vi "RT Driver VI.vi"(7 "Operation":T1, 11 "Device Reference in":T2 format="%.0x") -> (0 "Error Code":i32)   [LabVIEW 2020, in "FPGA Addon Engine.lvlib"]
uses:
  FPGA Addon Engine.lvlib
  <vilib>/NI VeriStand/Custom Device API/Custom Device Item Ref.ctl
  <vilib>/NI VeriStand/Custom Device API/Hardware Interface Driver VI Operation.ctl
  <vilib>/NI/NIVS Inline Async API/_VS Inline Async API/VS Inline Async API/Types/Error Handling Settings.ctl
  <vilib>/NI/NIVS Inline Async API/_VS Inline Async API/VS Inline Async API/VS Inline Async API.lvclass/VS Inline Async API.ctl
  <vilib>/NI/NIVS Inline Async API/_Data Access Engine/Data Access Engine/Data Access Engine.lvclass/Data Access Engine.ctl
  <vilib>/NI/NIVS Inline Async API/_Data Access Engine/Access Type Classes/Write/Write.lvclass/Write.ctl
  <vilib>/NI/NIVS Inline Async API/_Data Access Engine/Access Type Classes/ReadWrite/ReadWrite.lvclass/ReadWrite.ctl
  Addon Shared/SubVIs/FPGA Settings.vi
  SubVIs/Initialize Scalar Datatypes and Refs.vi
  <vilib>/NI/NIVS Inline Async API/_Data Access Engine/Data Access Engine/Methods/Data.Engine.Read Data from HW.vi
  <vilib>/NI/NIVS Inline Async API/_VS Inline Async API/Error Handling Process/SubVIs/Error.GetError.vi
  <vilib>/NI/NIVS Inline Async API/_Data Access Engine/Access Type Classes/ReadWrite/ReadWrite.EngineData.vi
  <vilib>/NI/NIVS Inline Async API/_Data Access Engine/Access Type Classes/Write/Write.EngineData.vi
  <vilib>/NI VeriStand/Custom Device API/NI VeriStand - Get Channel Value by Data Reference.vi
  <vilib>/NI VeriStand/Custom Device API/NI VeriStand - Set Channel Value by Data Reference.vi
  <vilib>/Utility/config.llb/Open Config Data.vi
  <vilib>/Utility/config.llb/Get Key Names.vi
  <vilib>/Utility/config.llb/Write Key.vi
  <vilib>/Utility/config.llb/Write Key (I32).vi
  <vilib>/Utility/config.llb/Close Config Data.vi
  Addon Shared/SubVIs/Constants.vi
  <vilib>/NI VeriStand/Custom Device API/NI VeriStand - Get Item Property.vi
  <vilib>/NI VeriStand/Custom Device API/Get Item Property (Variant).vi
  <vilib>/NI VeriStand/Custom Device API/Get Item Property (Dependent File).vi
  <vilib>/NI VeriStand/Custom Device API/Get Item Property (Path).vi
  <vilib>/NI VeriStand/Custom Device API/Get Item Property (String).vi
  <vilib>/NI VeriStand/Custom Device API/Get Item Property (Boolean).vi
  <vilib>/NI VeriStand/Custom Device API/NI VeriStand - Set Item Property.vi
  <vilib>/NI VeriStand/Custom Device API/Set Item Property (Path).vi
  <vilib>/NI VeriStand/Custom Device API/Set Item Property (String).vi
  <vilib>/NI VeriStand/Custom Device API/Set Item Property (Boolean).vi
  APIs/FPGA Register IO/Utilities/Open FPGA Session.vi
  SubVIs/Initialize Input DMA Refs.vi
  SubVIs/Initialize Output DMA Refs.vi
  SubVIs/Initialize Scalar Datatype Classes.vi
  <vilib>/Utility/SystemLogging/Write to System Log.vi
  <vilib>/Utility/error.llb/Error Cluster From Error Code.vi
  <vilib>/RVI Host/nirviSupport.llb/nirviErrorClusterFromErrorCode.vi
  <vilib>/rvi/errors/niLvFpgaAdjustHostInterfaceError.vi
  <vilib>/NI VeriStand/Custom Device API/Global Data Refs.vi
  <vilib>/FPGAPlugInAG/Dynamic/niLvFpga_Close_Dynamic.vi
  <vilib>/NI VeriStand/Custom Device Waveform API/Multiple Waveforms Write (DBL)/Multiple Waveforms Write (DBL).lvclass
  <vilib>/NI VeriStand/Custom Device Waveform API/Single Waveform Read (DBL)/Single Waveform Read (DBL).lvclass
  <vilib>/NI/NIVS Inline Async API/_VS Inline Async API/VS Inline Async API/VS Inline Async API.lvclass
  <vilib>/rvi/interface/nirviMethod/nirviMethod.xnode
  <vilib>/rvi/interface/nirviCloseFPGA/nirviCloseFPGA.xnode
  <vilib>/NI VeriStand/Custom Device API/Custom Device API.lvlib
  <vilib>/rvi/interface/nirviMethod/StockFPGA_InlinedMethodWaitForSingleIRQ.vi
  <vilib>/FPGAPlugInAG/Dynamic/niLvFpga_WaitOnIrq_Dynamic.vi
  <vilib>/FPGAPlugInAG/Dynamic/niLvFpga_AcknowledgeIrq_Dynamic.vi
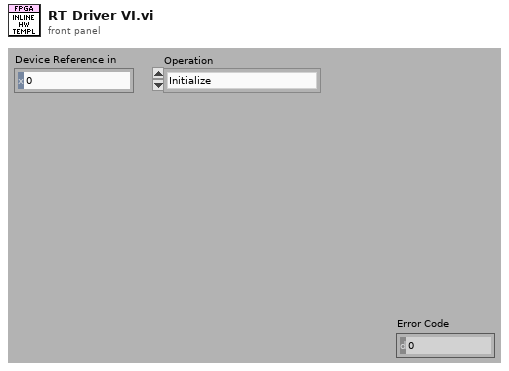
[diagram p1: front panel]
types:
  T1 = typedef "Custom Device API.lvlib/Hardware Interface Driver VI Operation.ctl" = enum16{"Initialize", "Start", "Read Data from HW", "Write Data to HW", "Close"}
  T2 = typedef "Custom Device API.lvlib/Custom Device Item Ref.ctl" = u64
  T3 = typedef "FPGA Addon Engine.lvlib/State Variables.ctl" = cluster{"FPGA Ref":refnum<k20>, "IncomingRegisters.Refs":T4[], "IncomingDMA.Refs":T7[], "OutgoingRegisters.Refs":T4[], "OutgoingDMA.Refs":T12[], "Compiled":T14}
  T4 = typedef "FPGA Addon Engine.lvlib/Register Settings.ctl" = cluster{"Name":string, "Data Type":T5, "session":u32, "Scalar Type":T6, "Index":i32, "Length":i32, "attributes":variant, "default value":variant}
  T5 = typedef "FPGA Addon Shared.lvlib/FPGA Addon Data Type.ctl" = enum8{"<Null>", "I8", "I16", "I32", "I64", "U8", "U16", "U32", "U64", "SGL", "Boolean", "Analog PWM In Settings", "Analog PWM In", "Digital PWM In Settings", "Digital PWM In", "Digital PWM Out", "Sine Out", "FXP", "FXP+/-24.5", "FXP+/-16.5", "FXP+/-32.8", "FXP+/-64.32", "FXP+/-16.7", "FXP+/-20.5", "FXP+/-27.5", "FXP+/-32.16", "FXP+16.3", "FXP+18.3", "Digital Static In", "Digital Static Out", "Digital Static In Settings", "Digital WSS Out", "Quad Encoder Settings", "Quad Encoder In", "Group"}
  T6 = typedef "FPGA Addon Shared.lvlib/Scalar Type.ctl" = enum16{"Standard", "Bitpacked"}
  T7 = typedef "FPGA Addon Engine.lvlib/DMA Input References.ctl" = cluster{"Addon Name":string, "Waveform Ref":refnum<class "Multiple Waveforms Write (DBL).lvclass">, "DMA Name":string, "DMA Settings":T8, "Refs":T11}
  T8 = typedef "FPGA Addon Shared.lvlib/DMA Settings.ctl" = cluster{"Number of Channels":u8, "Delacing Scheme":T9, "Update Rate":u32, "dt":dbl, "Mode":T10, "Number of Samples":u32, "DMA Host Buffer":u32}
  T9 = typedef "FPGA Addon Shared.lvlib/Delacing Scheme.ctl" = enum8{"Interleaved", "Bitpacked"}
  T10 = typedef "FPGA Addon Shared.lvlib/DMA Acquisition Mode.ctl" = enum8{"Continuous", "Triggered Finite"}
  T11 = typedef "FPGA Addon Engine.lvlib/DMA Input Refs.ctl" = cluster{"Data Type":T5, "DMA_SGL":refnum<k20>, "DMA_U64":refnum<k20>, "DMA_I64":refnum<k20>, "DMA_FXP+/-32.8":refnum<k20>, "DMA_FXP+/-64.32":refnum<k20>, "DMA_U32":refnum<k20>, "DMA_U16":refnum<k20>, "DMA_U8":refnum<k20>, "DMA_I32":refnum<k20>, "DMA_I16":refnum<k20>, "DMA_I8":refnum<k20>, "DMA_FXP+/-32.16":refnum<k20>}
  T12 = typedef "FPGA Addon Engine.lvlib/DMA Output References.ctl" = cluster{"Addon Name":string, "Waveforms":refnum<class "Single Waveform Read (DBL).lvclass">[], "DMA Name":string, "Refs":T13}
  T13 = typedef "FPGA Addon Engine.lvlib/DMA Output Refs.ctl" = cluster{"Data Type":T5, "DMA_SGL":refnum<k20>, "DMA_U64":refnum<k20>, "DMA_I64":refnum<k20>, "DMA_FXP+/-32.8":refnum<k20>, "DMA_FXP+/-64.32":refnum<k20>, "DMA_U32":refnum<k20>, "DMA_U16":refnum<k20>, "DMA_U8":refnum<k20>, "DMA_I32":refnum<k20>, "DMA_I16":refnum<k20>, "DMA_I8":refnum<k20>, "DMA_FXP+/-32.16":refnum<k20>}
  T14 = typedef "FPGA Addon Shared.lvlib/Compiled.Settings.ctl" = cluster{"Name":string, "IncomingRegisters.Settings":T15[], "IncomingRegisters.Refs":cluster{"Refs":T17[], "Values":dbl[]}, "OutgoingRegisters.Settings":T15[], "OutgoingRegisters.Refs":cluster{"Refs":T17[], "Values":dbl[]}, "Incoming.Size":i32, "Outgoing.Size":i32, "IncomingDMA.Settings":T19[], "OutgoingDMA.Settings":T19[], "FPGA.Settings":T21, "Target.Type":T22}
  T15 = typedef "FPGA Addon Shared.lvlib/Compiled.RegisterSettings.ctl" = cluster{"Scalar Type":T6, "Index":i32, "Length":i32, "Register":T16}
  T16 = typedef "FPGA Addon Shared.lvlib/Register Information.ctl" = cluster{"Name":string, "Data Type":T5, "Default Value":variant, "Attributes":variant}
  T17 = typedef "Custom Device API.lvlib/Block Data Reference.ctl" = cluster{"Data Reference":T18, "Offset":u64, "Length":u64}
  T18 = typedef "Custom Device API.lvlib/Data Reference.ctl" = i32
  T19 = typedef "FPGA Addon Shared.lvlib/Compiled.DMASettings.ctl" = cluster{"Name":string, "Data Type":T5, "DMA.Settings":T8, "DMA.VSRefs":T20[]}
  T20 = typedef "Custom Device API.lvlib/Waveform Data Reference.ctl" = i32
  T21 = typedef "FPGA Addon Shared.lvlib/FPGA Settings.ctl" = cluster{"Bitfile path":path, "RIO Device Address":string, "Group":bool}
  T22 = typedef "Custom Device API.lvlib/Custom Device Target Type.ctl" = enum16{"PharLap", "VxWorks", "Windows", "Linux_32_ARM", "Linux_x64"}
  T23 = cluster{"Vars":T3, "Async?":bool, "Async":refnum<class "VS Inline Async API.lvclass">}
  T24 = typedef "VS Inline Async API.lvlib/VS Inline Async API.lvclass/Error Handling Settings.ctl" = cluster{"Write to SystemLog (F)":bool}
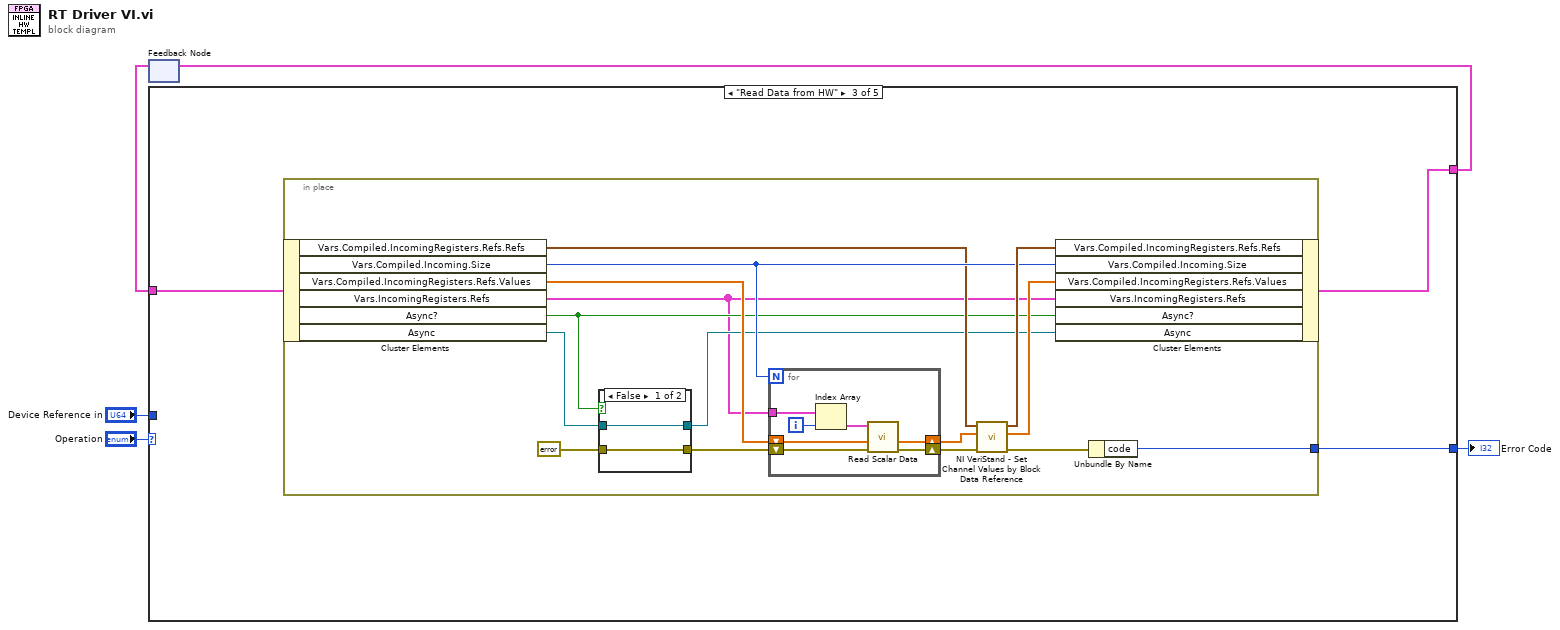
[diagram p0: block diagram]
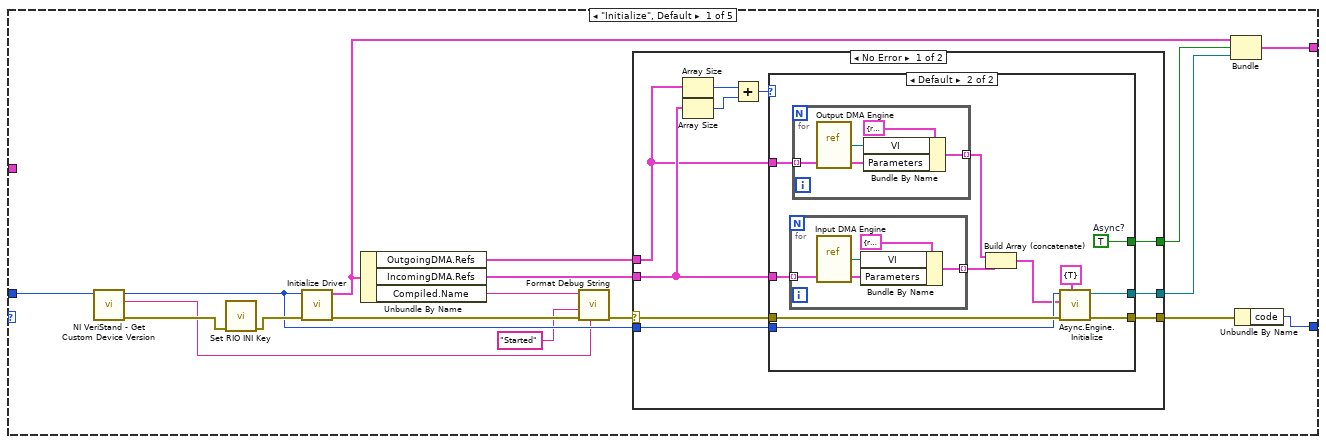
[diagram p2: hidden frame]
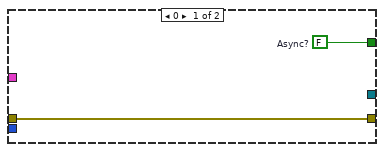
[diagram p3: hidden frame]
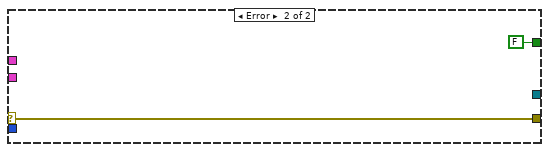
[diagram p4: hidden frame]
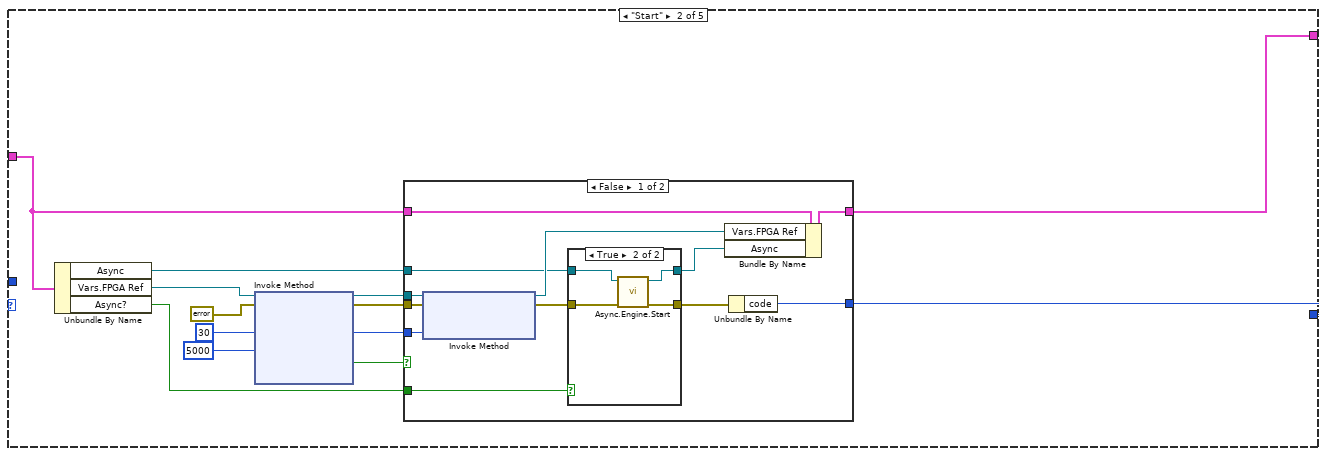
[diagram p5: hidden frame]
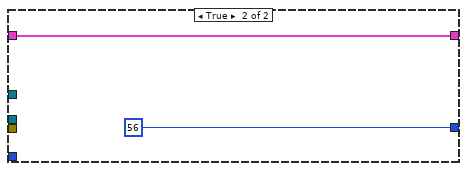
[diagram p7: hidden frame]
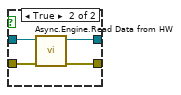
[diagram p8: hidden frame]
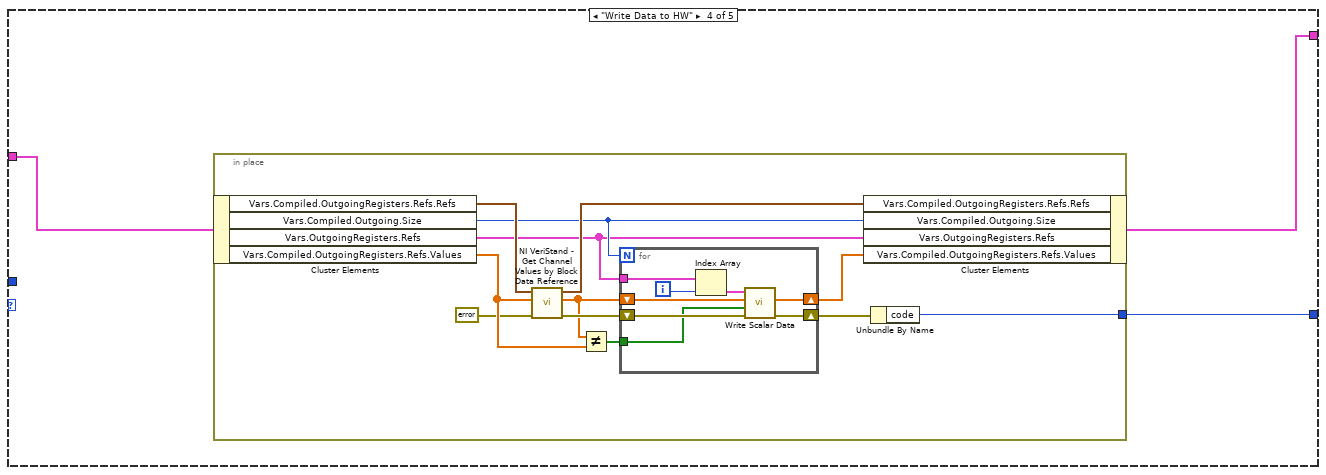
[diagram p9: hidden frame]
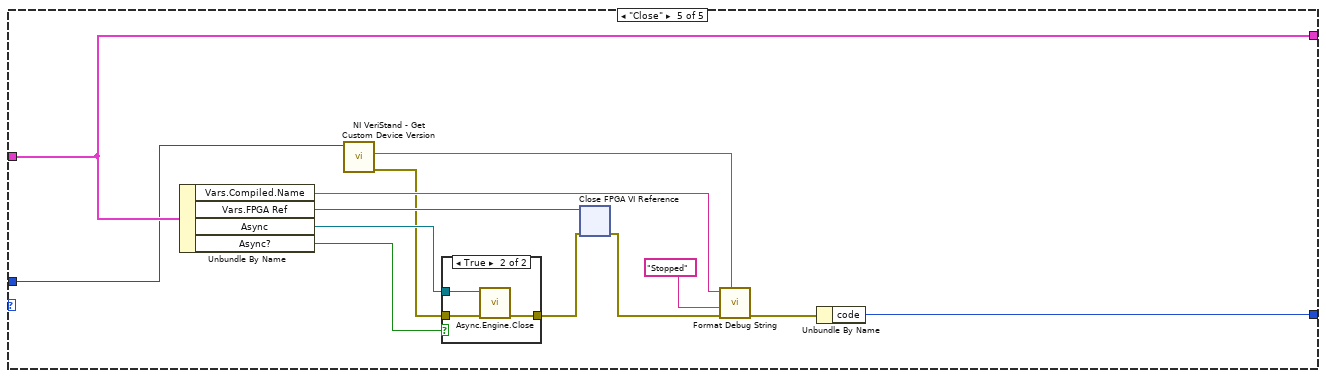
[diagram p10: hidden frame]
diagram:
  n1 = feedback #1() -> (w3:T23)  [unwired: 1 out]
  n2 = case shown="\"Read Data from HW\"" "Operation" {
    tunnel: [w22 w65 w90 w120 w153] -> w4
    tunnel: w3 -> [_ w66 w88 w121 w153]
    tunnel: "Device Reference in" -> [w12 _ _ _ w148]
    tunnel: [w21 w67 w89 w119 w154] -> w1
    frame "Initialize", Default {
      n3 = call <vilib>:"NI VeriStand - Get Custom Device Version.vi"("Device Ref in"=w12) -> ("error out"=w13:errorcluster, "Value"=w9:string, "Device Ref out"=w11:T2)  [unwired: 8 in]
      n4 = call "Set RIO INI Key.vi"("error in (no error)"=w13) -> ("error out"=w20:errorcluster)  [unwired: 10 in]
      n5 = call "Initialize Driver.vi"("error in (no error)"=w20, "Section Ref in"=w11) -> ("error out"=w10:errorcluster, "Vars"=w14:T3)  [unwired: 8 in]
      n6 = Unbundle By Name(w14) -> ("OutgoingDMA.Refs"=w16:T12[], "IncomingDMA.Refs"=w17:T7[], "Compiled.Name"=w8:string)
      n7 = call "Format Debug String.vi"("Version"=w9, "error in (no error)"=w10, "State"="Started" ("string"), "Name"=w8) -> ("error out"=w6:errorcluster)  [unwired: 7 in]
      n8 = case shown="No Error" w6 {
        selector: w6 -> [w23 w55]
        tunnel: [w32 w55] -> w19
        tunnel: [w31 _] -> w18
        tunnel: w17 -> [w30 _]
        tunnel: w16 -> [w29 _]
        tunnel: [w25 FALSE ("Async?")] -> w15
        tunnel: w11 -> [w24 _]
        frame No Error {
          n9 = Array Size(array=w29) -> (size(s)=w28:i32)
          n10 = Array Size(array=w30) -> (size(s)=w27:i32)
          n11 = Add(x=w28, y=w27) -> (x+y=w26:i32)
          n12 = case shown="Default" w26 {
            tunnel: w23 -> [w34 w42]
            tunnel: [w34 w41] -> w32
            tunnel: [_ w40] -> w31
            tunnel: w30 -> [_ w38]
            tunnel: w29 -> [_ w45]
            tunnel: [w33 w43] -> w25
            tunnel: w24 -> [_ w39]
            frame 0 {
              w33 = FALSE  # Async?
            }
            frame Default {
              w43 = TRUE  # Async?
              n13 = for {
                tunnel: w38 -> [w46] mode=indexing
                tunnel: [w48] -> w37 mode=indexing
                n14 = vi-ref "Input DMA Engine.vi"() -> (w47:refnum<vi>)
                n15 = Bundle By Name(cluster=cluster{"VI":refnum<vi>, "Parameters":variant} {"VI"=refnum, "Parameters"=variant} ("Process"), "VI"=w47, "Parameters"=w46) -> (w48:cluster{"VI":refnum<vi>, "Parameters":variant})
              }
              n16 = for {
                tunnel: w45 -> [w52] mode=indexing
                tunnel: [w51] -> w44 mode=indexing
                n17 = vi-ref "Output DMA Engine.vi"() -> (w50:refnum<vi>)
                n18 = Bundle By Name(cluster=cluster{"VI":refnum<vi>, "Parameters":variant} {"VI"=refnum, "Parameters"=variant} ("Process"), "VI"=w50, "Parameters"=w52) -> (w51:cluster{"VI":refnum<vi>, "Parameters":variant})
              }
              n19 = Build Array (concatenate)(w44, w37) -> (w36:cluster{"VI":refnum<vi>, "Parameters":variant}[])
              n20 = call <vilib>:"Async.Engine.Initialize.vi"("Error Log Settings"=T24 {"Write to SystemLog (F)"=TRUE}, "error in (no error)"=w42, "Processes"=w36, "Custom Device Ref"=w39) -> ("error out"=w41:errorcluster, "Async"=w40:refnum<class "VS Inline Async API.lvclass">)  [unwired: 6 in]
            }
          }
        }
        frame Error {
        }
      }
      n21 = Bundle("Vars"=w14, "Async?"=w15, "Async"=w18) -> (w22:T23)  [unwired: 1 out]
      n22 = Unbundle By Name(w19) -> ("code"=w21:i32)
    }
    frame "Start" {
      w61 = 30 ("IRQ Number(s)")
      n23 = Unbundle By Name(w66) -> ("Async"=w57:refnum<class "VS Inline Async API.lvclass">, "Vars.FPGA Ref"=w64:refnum<k20>, "Async?"=w59:bool)
      n24 = xnode "Invoke Method"("FPGA VI Reference In"=w64, "error in"=errorcluster {"status"=FALSE, "code"=0, "source"=""}, "IRQ Number(s)"=w61, "Timeout (ms)"=5000) -> ("FPGA VI Reference Out"=w63:refnum<k20>, "error out"=w62:errorcluster, "Timed Out"=w58:bool)  [unwired: 1 out]
      n25 = case shown="False" w58 {
        tunnel: [w79 56 ("code")] -> w67
        tunnel: w66 -> [w78 w87]
        tunnel: [w77 w87] -> w65
        tunnel: w63 -> [w76 _]
        tunnel: w62 -> [w75 _]
        tunnel: w61 -> [w74 _]
        tunnel: w59 -> [w71 _]
        tunnel: w57 -> [w70 _]
        frame False {
          n26 = xnode "Invoke Method"("FPGA VI Reference In"=w76, "error in"=w75, "IRQ Number(s)"=w74) -> ("FPGA VI Reference Out"=w73:refnum<k20>, "error out"=w68:errorcluster)
          n27 = case shown="True" w71 {
            tunnel: w68 -> [w81 w85]
            tunnel: [w81 w84] -> w72
            tunnel: w70 -> [w80 w83]
            tunnel: [w80 w82] -> w69
            frame False {
            }
            frame True {
              n28 = call <vilib>:"Async.Engine.Start.vi"("error in (no error)"=w85, "VS Inline Async API in"=w83) -> ("error out"=w84:errorcluster, "VS Inline Async API out"=w82:refnum<class "VS Inline Async API.lvclass">)  [unwired: 8 in]
            }
          }
          n29 = Bundle By Name(cluster=w78, "Vars.FPGA Ref"=w73, "Async"=w69) -> (w77:T23)
          n30 = Unbundle By Name(w72) -> ("code"=w79:i32)
        }
        frame True {
        }
      }
    }
    frame "Read Data from HW" {
      n31 = in-place {
        in-place-border: [w97] -> w89
        n32 = in-place-cluster #2(w88) -> ("Vars.Compiled.IncomingRegisters.Refs.Refs"=w99:T17[], "Vars.Compiled.Incoming.Size"=w101:i32, "Vars.Compiled.IncomingRegisters.Refs.Values"=w105:dbl[], "Vars.IncomingRegisters.Refs"=w91:T4[], "Async?"=w93:bool, "Async"=w95:refnum<class "VS Inline Async API.lvclass">)
        n33 = case shown="False" w93 {
          tunnel: w95 -> [w107 w111]
          tunnel: [w106 w110] -> w96
          tunnel: [w107 w109] -> w94
          tunnel: errorcluster {"status"=FALSE, "code"=0, "source"=""} ("error in") -> [w106 w108]
          frame False {
          }
          frame True {
            n34 = call <vilib>:"Async.Engine.Read Data from HW.vi"("error in"=w108, "Async in"=w111) -> ("error out"=w110:errorcluster, "Async out"=w109:refnum<class "VS Inline Async API.lvclass">)  [unwired: 8 in]
          }
        }
        n35 = for {
          N: w101 -> [_]
          shift-right: [w112] -> w102
          shift-left: w105 -> [w113]
          shift-right: [w116] -> w100
          shift-left: w96 -> [w117]
          tunnel: w91 -> [w118]
          i -> [w114]
          n36 = Index Array(array=w118, index=w114) -> (element=w115:T4)
          n37 = call "Read Scalar Data.vi"("error in (no error)"=w117, "Values"=w113, "Cluster"=w115) -> ("error out"=w116:errorcluster, "Values"=w112:dbl[])  [unwired: 7 in]
        }
        n38 = call <vilib>:"NI VeriStand - Set Channel Values by Block Data Reference.vi"("error in (no error)"=w100, "Values Array in"=w102, "Block Data Ref"=w99) -> ("error out"=w98:errorcluster, "Values Array out"=w103:dbl[], "Block Data Ref dup"=w104:T17[])  [unwired: 6 in]
        n39 = in-place-cluster #2("Vars.Compiled.IncomingRegisters.Refs.Refs"=w104, "Vars.Compiled.Incoming.Size"=w101, "Vars.Compiled.IncomingRegisters.Refs.Values"=w103, "Vars.IncomingRegisters.Refs"=w91, "Async?"=w93, "Async"=w94) -> (w90:T23)
        n40 = Unbundle By Name(w98) -> ("code"=w97:i32)
      }
    }
    frame "Write Data to HW" {
      n41 = in-place {
        in-place-border: [w127] -> w119
        n42 = in-place-cluster #3(w121) -> ("Vars.Compiled.OutgoingRegisters.Refs.Refs"=w133:T17[], "Vars.Compiled.Outgoing.Size"=w129:i32, "Vars.OutgoingRegisters.Refs"=w122:T4[], "Vars.Compiled.OutgoingRegisters.Refs.Values"=w125:dbl[])
        n43 = call <vilib>:"NI VeriStand - Get Channel Values by Block Data Reference.vi"("error in (no error)"=errorcluster {"status"=FALSE, "code"=0, "source"=""} ("error in"), "Values Array in"=w125, "Block Data Ref"=w133) -> ("error out"=w130:errorcluster, "Values Array out"=w126:dbl[], "Block Data Ref dup"=w132:T17[])  [unwired: 6 in]
        n44 = Not Equal?(x=w126, y=w125) -> (x != y?=w124:bool[])
        n45 = for {
          N: w129 -> [_]
          shift-right: [w135] -> w131
          shift-left: w126 -> [w140]
          shift-right: [w136] -> w128
          shift-left: w130 -> [w141]
          tunnel: w124 -> [w134]
          tunnel: w122 -> [w139]
          i -> [w137]
          n46 = Index Array(array=w139, index=w137) -> (element=w138:T4)
          n47 = call "Write Scalar Data.vi"("error in (no error)"=w141, "Changed?"=w134, "Values"=w140, "Cluster"=w138) -> ("error out"=w136:errorcluster, "Values"=w135:dbl[])  [unwired: 6 in]
        }
        n48 = in-place-cluster #3("Vars.Compiled.OutgoingRegisters.Refs.Refs"=w132, "Vars.Compiled.Outgoing.Size"=w129, "Vars.OutgoingRegisters.Refs"=w122, "Vars.Compiled.OutgoingRegisters.Refs.Values"=w131) -> (w120:T23)
        n49 = Unbundle By Name(w128) -> ("code"=w127:i32)
      }
    }
    frame "Close" {
      n50 = Unbundle By Name(w153) -> ("Vars.Compiled.Name"=w143:string, "Vars.FPGA Ref"=w151:refnum<k20>, "Async"=w149:refnum<class "VS Inline Async API.lvclass">, "Async?"=w150:bool)
      n51 = call <vilib>:"NI VeriStand - Get Custom Device Version.vi"("Device Ref in"=w148) -> ("error out"=w142:errorcluster, "Value"=w144:string)  [unwired: 8 in, 1 out]
      n52 = case shown="True" w150 {
        tunnel: [w155 w158] -> w152
        tunnel: w149 -> [_ w157]
        tunnel: w142 -> [w155 w156]
        frame False {
        }
        frame True {
          n53 = call <vilib>:"Async.Engine.Close.vi"("error in (no error)"=w156, "Async in"=w157) -> ("error out"=w158:errorcluster)  [unwired: 8 in, 1 out]
        }
      }
      n54 = xnode "Close FPGA VI Reference"("FPGA VI Reference In"=w151, "error in"=w152) -> ("error out"=w145:errorcluster)
      n55 = call "Format Debug String.vi"("Version"=w144, "error in (no error)"=w145, "State"="Stopped" ("string"), "Name"=w143) -> ("error out"=w146:errorcluster)  [unwired: 7 in]
      n56 = Unbundle By Name(w146) -> ("code"=w154:i32)
    }
  }
  "Error Code" <- w1
  n57 = feedback-in #1(w4) -> ()
